vi "set-locking.vi"(10 "locking":enum16{"off", "reg a", "reg b"}(ring)) -> (0 "error out":errorcluster)   [LabVIEW 2014]
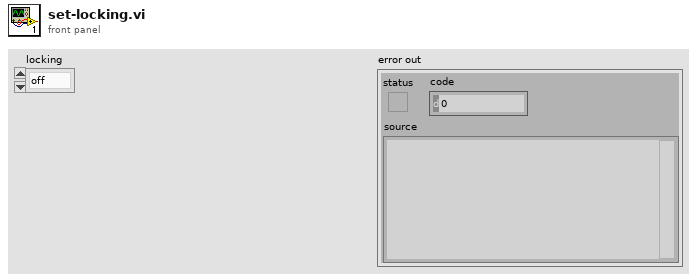
[diagram p1: front panel]
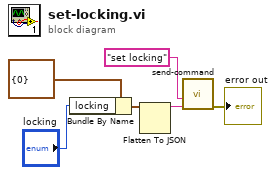
[diagram p0: block diagram]
diagram:
  n1 = Bundle By Name(cluster=cluster{"locking":u8} {"locking"=0}, "locking"="locking") -> (w1:cluster{"locking":u8})
  n2 = Flatten To JSON(anything=w1) -> (JSON string=w5:string)  [unwired: 2 in, 1 out]
  n3 = call "send-command.vi"("parameters"=w5, "command"="set locking") -> ("error out"=→"error out":errorcluster)  [unwired: 8 in, 1 out]
